vi "Icon_Build Template array.vi"(8 "Error":errorcluster, 11 "Set Array":T2[](array[typedef]) {"Format"."Icon Sizing"."Rows" min=1 max=5 step=1; "Format"."Icon Sizing"."Width" min=7 max=32 step=1}) -> (0 "Error Out":errorcluster, 3 "Template Array Out":T1[](array[typedef]))   [LabVIEW 2009]
doc: "Builds a template icon for each color set"
uses:
  Controls/Cluster/Cluster_Format Storage.ctl
  Controls/String_Picture/STRING_Line Display.ctl
  Controls/Cluster/Cluster_Icon Format.ctl
  Controls/Cluster/Cluster_Icon Color Set.ctl
  Controls/Enum/ENUM_Frame Template Select.ctl
  Controls/Cluster/Cluster_Sizing Data.ctl
  Controls/Enum/ENUM_Icon Sizing.ctl
  Controls/Enum/RBENUM_Icon Position.ctl
  Controls/String_Picture/Picture_Icon.ctl
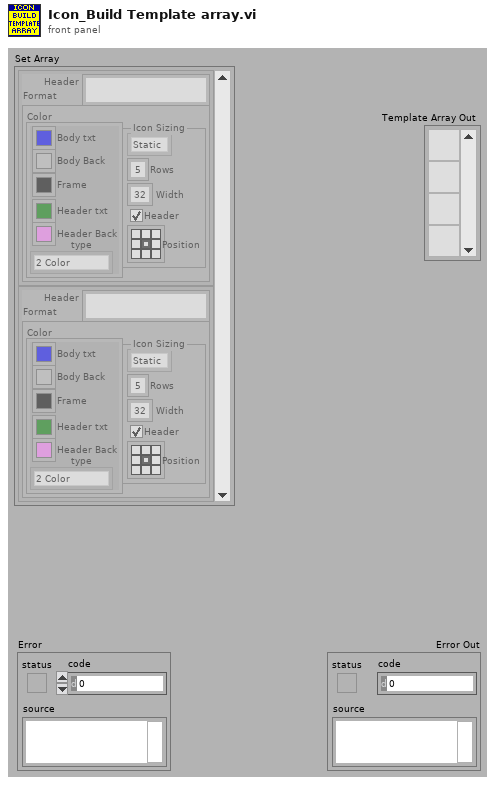
[diagram p1: front panel]
types:
  T1 = typedef "Picture_Icon.ctl" = picture
  T2 = typedef "Cluster_Format Storage.ctl" = cluster{"Header":T3, "Format":T4}
  T3 = typedef "STRING_Line Display.ctl" = string
  T4 = typedef "Cluster_Icon Format.ctl" = cluster{"Color":T5, "Icon Sizing":T7}
  T5 = typedef "Cluster_Icon Color Set.ctl" = cluster{"Body txt":u32, "Body Back":u32, "Frame":u32, "Header txt":u32, "Header Back":u32, "type":T6}
  T6 = typedef "ENUM_Frame Template Select.ctl" = enum16{"2 Color", "5 Color"}
  T7 = typedef "Cluster_Sizing Data.ctl" = cluster{"Rule":T8, "Header":bool, "Rows":u32, "Width":u32, "Position":T9}
  T8 = typedef "ENUM_Icon Sizing.ctl" = enum16{"Static", "Auto"}
  T9 = typedef "RBENUM_Icon Position.ctl" = enum32{"LFT-TOP", "MID-TOP", "RGT-TOP", "LFT-CTR", "MID-CTR", "RGT-CTR", "LFT-BOT", "MID-BOT", "RGT-BOT"}
  T10 = typedef "Cluster_Icon Data.ctl" = cluster{"Header":T3, "Body":T11, "ImageData":T12, "New Icon":T1, "Line Status":bool[], "Format":T4}
  T11 = typedef "String Array_Body Text.ctl" = T3[]
  T12 = typedef "Cluster_Image Data.ctl" = cluster{"image type":i32, "image depth":i32, "image":u8[], "mask":u8[], "colors":u32[], "Rectangle":T13}
  T13 = typedef "CLuster_Selectoin Box.ctl" = cluster{"left":i16, "top":i16, "right":i16, "bottom":i16}
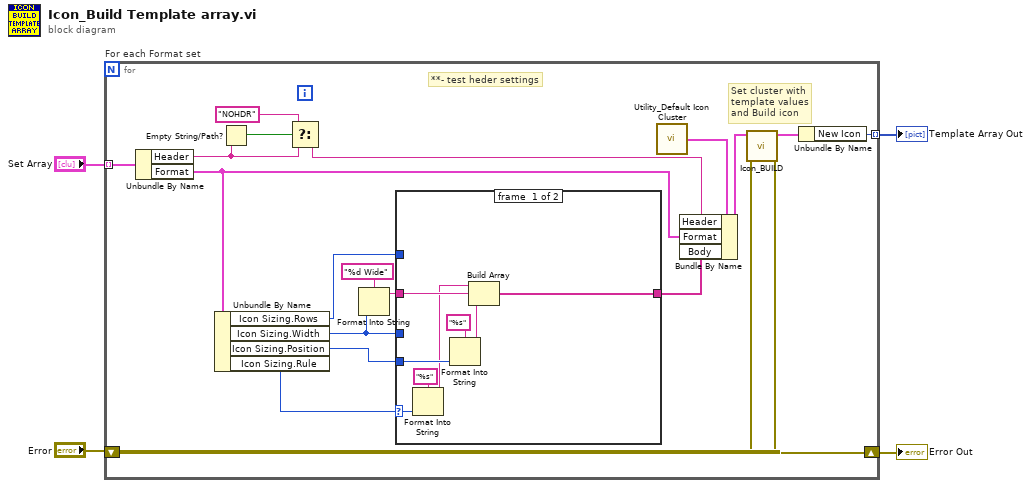
[diagram p0: block diagram]
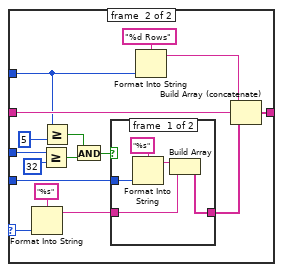
[diagram p2: hidden frame]
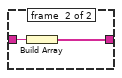
[diagram p3: hidden frame]
diagram:
  n1 = for "For each Format set" {
    shift-right: [w21] -> w3
    shift-left: "Error" -> [w22]
    tunnel: "Set Array" -> [w18] mode=indexing
    tunnel: [w19] -> w2 mode=indexing
    # "**- test heder settings"
    # "Set cluster with\ntemplate values \nand Build icon"
    n2 = Unbundle By Name(w18) -> ("Header"=w7:T3, "Format"=w10:T4)
    n3 = Unbundle By Name(w10) -> ("Icon Sizing.Rows"=w14:u32, "Icon Sizing.Width"=w12:u32, "Icon Sizing.Position"=w13:T9, "Icon Sizing.Rule"=w11:T8)
    n4 = Empty String/Path?(string/path=w7) -> (empty?=w8:bool)
    n5 = Select(t=T3 "NOHDR", s=w8, f=w7) -> (s? t:f=w6:T3)
    n6 = Format Into String(format string="%d Wide", w12) -> (resulting string=w16:string)  [unwired: 2 in, 1 out]
    n7 = case shown="\"Auto\"" w11 {
      selector: w11 -> [w31 w47]
      tunnel: w14 -> [_ w38]
      tunnel: w16 -> [w30 w44]
      tunnel: [w29 w43] -> w15
      tunnel: w13 -> [w27 w42]
      tunnel: w12 -> [_ w40]
      frame #0 {
        n8 = Format Into String(format string="%s", w31) -> (resulting string=w24:string)  [unwired: 2 in, 1 out]
        n9 = Format Into String(format string="%s", w27) -> (resulting string=w26:string)  [unwired: 2 in, 1 out]
        n10 = Build Array(w24, w30, w26) -> (w29:string[])
      }
      frame #1 {
        n11 = Format Into String(format string="%s", w47) -> (resulting string=w33:string)  [unwired: 2 in, 1 out]
        n12 = Greater Or Equal?(x=w40, y=u32 32) -> (x >= y?=w35:bool)
        n13 = Greater Or Equal?(x=w38, y=u32 5) -> (x >= y?=w36:bool)
        n14 = And(x=w36, y=w35) -> (x .and. y?=w34:bool)
        n15 = case shown="False" w34 {
          tunnel: w42 -> [w51 _]
          tunnel: [w49 w53] -> w41
          tunnel: w33 -> [w48 w54]
          frame #0 {
            n16 = Format Into String(format string="%s", w51) -> (resulting string=w50:string)  [unwired: 2 in, 1 out]
            n17 = Build Array(w50, w48) -> (w49:string[])
          }
          frame #1 {
            n18 = Build Array(w54) -> (w53:string[])
          }
        }
        n19 = Format Into String(format string="%d Rows", w38) -> (resulting string=w32:string)  [unwired: 2 in, 1 out]
        n20 = Build Array (concatenate)(w32, w44, w41) -> (w43:string[])
      }
    }
    n21 = call "Utility_Default Icon Cluster.vi"() -> ("Default Cluster"=w9:T10)  [unwired: 2 in]
    n22 = Bundle By Name(cluster=w9, "Header"=w6, "Format"=w10, "Body"=w15) -> (w23:T10)
    n23 = call "Icon_BUILD.vi"("Error"=w22, "ICON Cluster"=w23) -> ("Error Out"=w21:errorcluster, "ICON Cluster Out"=w20:T10)  [unwired: 7 in, 1 out]
    n24 = Unbundle By Name(w20) -> ("New Icon"=w19:T1)
  }
  "Error Out" <- w3
  "Template Array Out" <- w2
